vi "isVariantEmpty.vi"(4 "Anything":variant) -> (1 "empty?":bool)   [LabVIEW 2009]
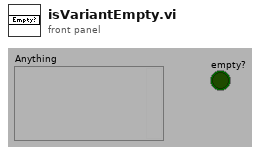
[diagram p1: front panel]
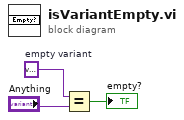
[diagram p0: block diagram]
diagram:
  w2 = variant  # empty variant
  n1 = Equal?(x=w2, y="Anything") -> (x = y?=→"empty?":bool)
